vi "parseStatus.vi"(8 "error in (no error)":errorcluster, 9 "timeout":bool=TRUE, 10 "Message":string, 11 "tcpExampleControler in":refnum<class "tcpExampleControler.lvclass">) -> (0 "error out":errorcluster, 2 "status":T1, 3 "tcpExampleControler out":refnum<class "tcpExampleControler.lvclass">)   [LabVIEW 2016, in "tcpExampleControler.lvclass"]
uses:
  tcpExampleControler.lvclass
  typedefs/deviceStatus.ctl
  typedefs/statusEnum.ctl
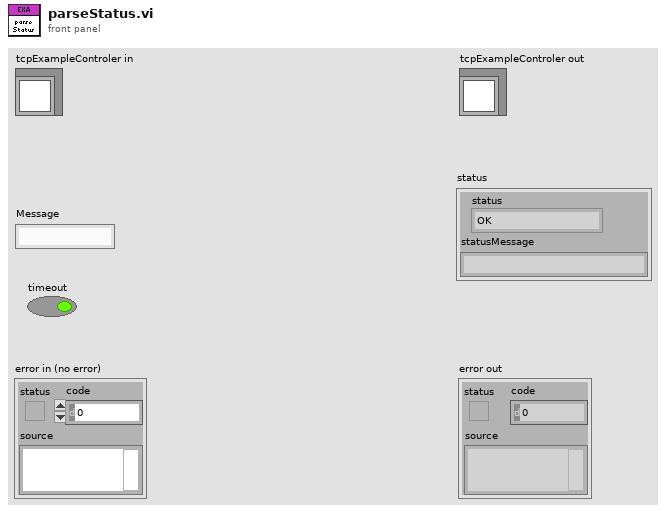
[diagram p1: front panel]
types:
  T1 = typedef "deviceStatus.ctl" = cluster{"status":T2, "statusMessage":string}
  T2 = typedef "statusEnum.ctl" = enum16{"OK", "TIMEOUT", "MSGERROR"}
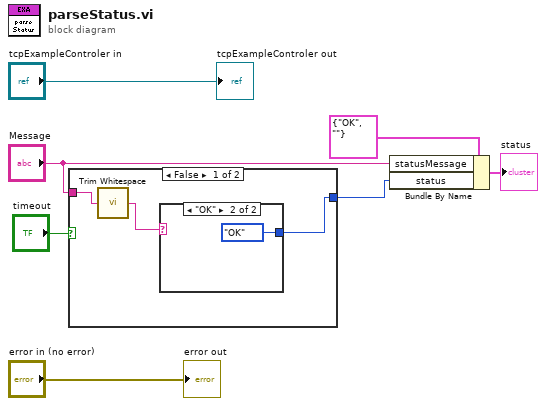
[diagram p0: block diagram]
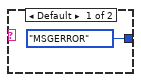
[diagram p2: hidden frame]
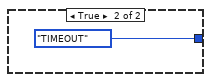
[diagram p3: hidden frame]
diagram:
  n1 = case shown="False" "timeout" {
    tunnel: [w10 statusEnum."TIMEOUT" ("status")] -> w2
    tunnel: "Message" -> [w8 _]
    frame False {
      n2 = call <vilib>:"Trim Whitespace.vi"("string"=w8) -> ("trimmed string"=w9:string)  [unwired: 1 in]
      n3 = case shown="\"OK\"" w9 {
        tunnel: [statusEnum."MSGERROR" ("status") statusEnum."OK" ("status")] -> w10
        frame Default {
        }
        frame "OK" {
        }
      }
    }
    frame True {
    }
  }
  n4 = Bundle By Name(cluster=T1 {"status"=enum."OK", "statusMessage"=""} ("status"), "statusMessage"="Message", "status"=w2) -> (→"status":T1)
  "error out" <- "error in (no error)"
  "tcpExampleControler out" <- "tcpExampleControler in"
